vi "programa 13.vi"() -> ()   [LabVIEW 2011]
panel:
  in  "stop":bool
  out "velocidad":i32(knob) scale=0.0..180.0
  in  "disminuir":bool
  in  "aumentar":bool
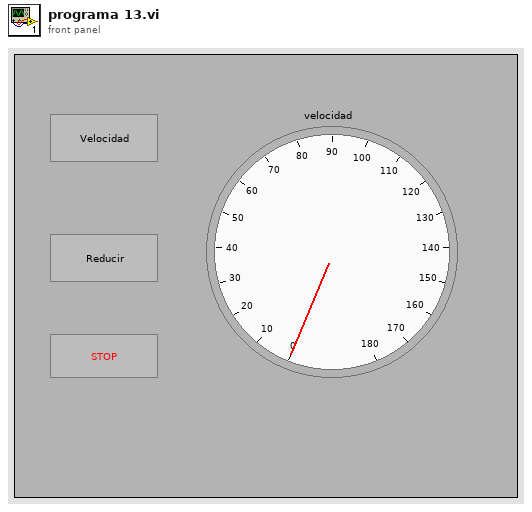
[diagram p1: front panel]
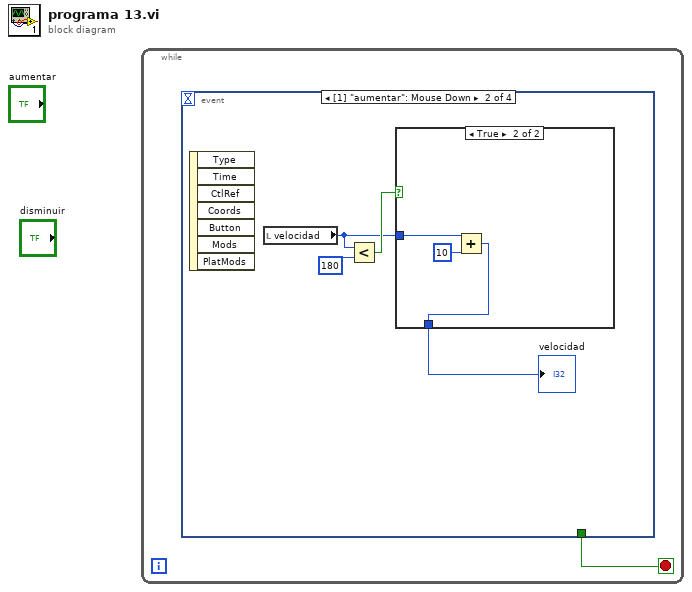
[diagram p0: block diagram]
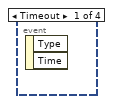
[diagram p2: hidden frame]
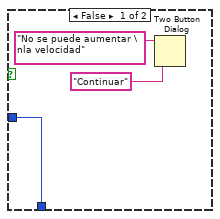
[diagram p3: hidden frame]
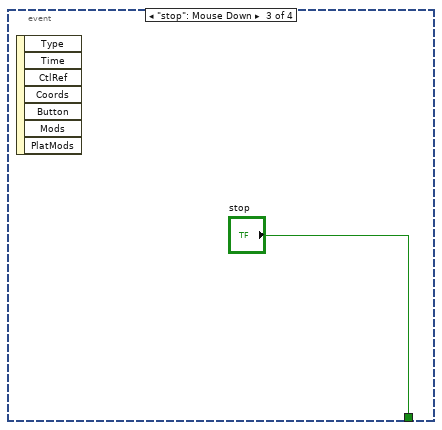
[diagram p4: hidden frame]
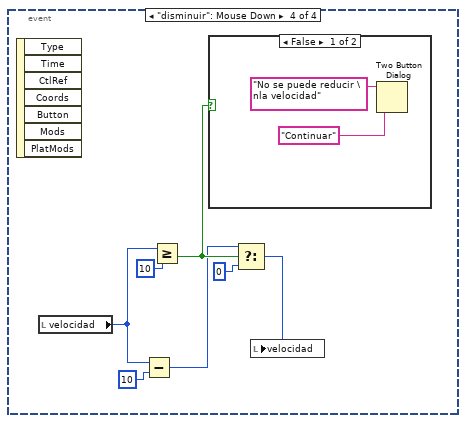
[diagram p5: hidden frame]
diagram:
  n1 = while {
    stop <- w1 stop-if-true
    n2 = event shown="[1] \"aumentar\": Mouse Down" {
      selector: _ -> [_ _ _ _]
      dyn-events: _ -> [_ _ _ _]
      timeout: _ -> [_ _ _ _]
      tunnel: [_ _ "stop" _] -> w1
      event Timeout {
        n3 = event-data() -> ()  [unwired: 1 in, 2 out]
      }
      event "aumentar": Mouse Down {
        n4 = event-data() -> ()  [unwired: 1 in, 7 out]
        n5 = local read "velocidad"() -> (w3:i32)
        n6 = Less?(x=w3, y=180) -> (x < y?=w4:bool)
        n7 = case shown="True" w4 {
          tunnel: w3 -> [w6 w10]
          tunnel: [w6 w9] -> w2
          frame False {
            n8 = Two Button Dialog(message="No se puede aumentar \nla velocidad", 1:"Continuar" ("F button name (\"Cancel\")")) -> ()  [unwired: 1 in, 1 out]
          }
          frame True {
            n9 = Add(x=w10, y=10) -> (x+y=w9:i32)
          }
        }
        "velocidad" <- w2
      }
      event "stop": Mouse Down {
        n10 = event-data() -> ()  [unwired: 1 in, 7 out]
      }
      event "disminuir": Mouse Down {
        n11 = event-data() -> ()  [unwired: 1 in, 7 out]
        n12 = local read "velocidad"() -> (w17:i32)
        n13 = Subtract(x=w17, y=10) -> (x-y=w13:i32)
        n14 = Greater Or Equal?(x=w17, y=10) -> (x >= y?=w15:bool)
        n15 = case shown="False" w15 {
          frame False {
            n16 = Two Button Dialog(message="No se puede reducir \nla velocidad", 1:"Continuar" ("F button name (\"Cancel\")")) -> ()  [unwired: 1 in, 1 out]
          }
          frame True {
          }
        }
        n17 = Select(t=w13, s=w15, f=0) -> (s? t:f=w16:i32)
        n18 = local write "velocidad"(w16) -> ()
      }
    }
  }
